vi "Controller Request Stop.vi"(7 "Sync Objects":T2, 8 "error in (no error)":errorcluster) -> (0 "error out":errorcluster)   [LabVIEW 2011, in "Controller VIs.lvlib"]
doc: "Requests the completion of all parallel loops running in the FOFB Controller. Sends a stop notification through the \"Stop Notifier\" and forces all blocking notifiers to be released."
uses:
  Controller VIs.lvlib
  Types Definitions/Type Synchronization Objects.ctl
  Types Definitions/Type Blocking Synchronization Objects.ctl
  Types Definitions/Type Monitoring Data.ctl
  Types Definitions/Type Operation Mode State.ctl
  Types Definitions/Type Diagnostics Data.ctl
  Types Definitions/Type CPU Loads Array.ctl
  Types Definitions/Type CPU Loads.ctl
  Types Definitions/Type Non-blocking Synchronization Objects.ctl
  Types Definitions/Type FOFB Variables.ctl
  Types Definitions/Type Actuation State.ctl
  Misc VIs.lvlib
  Type Definitions.lvlib
panel:
  out "Blocking":T1
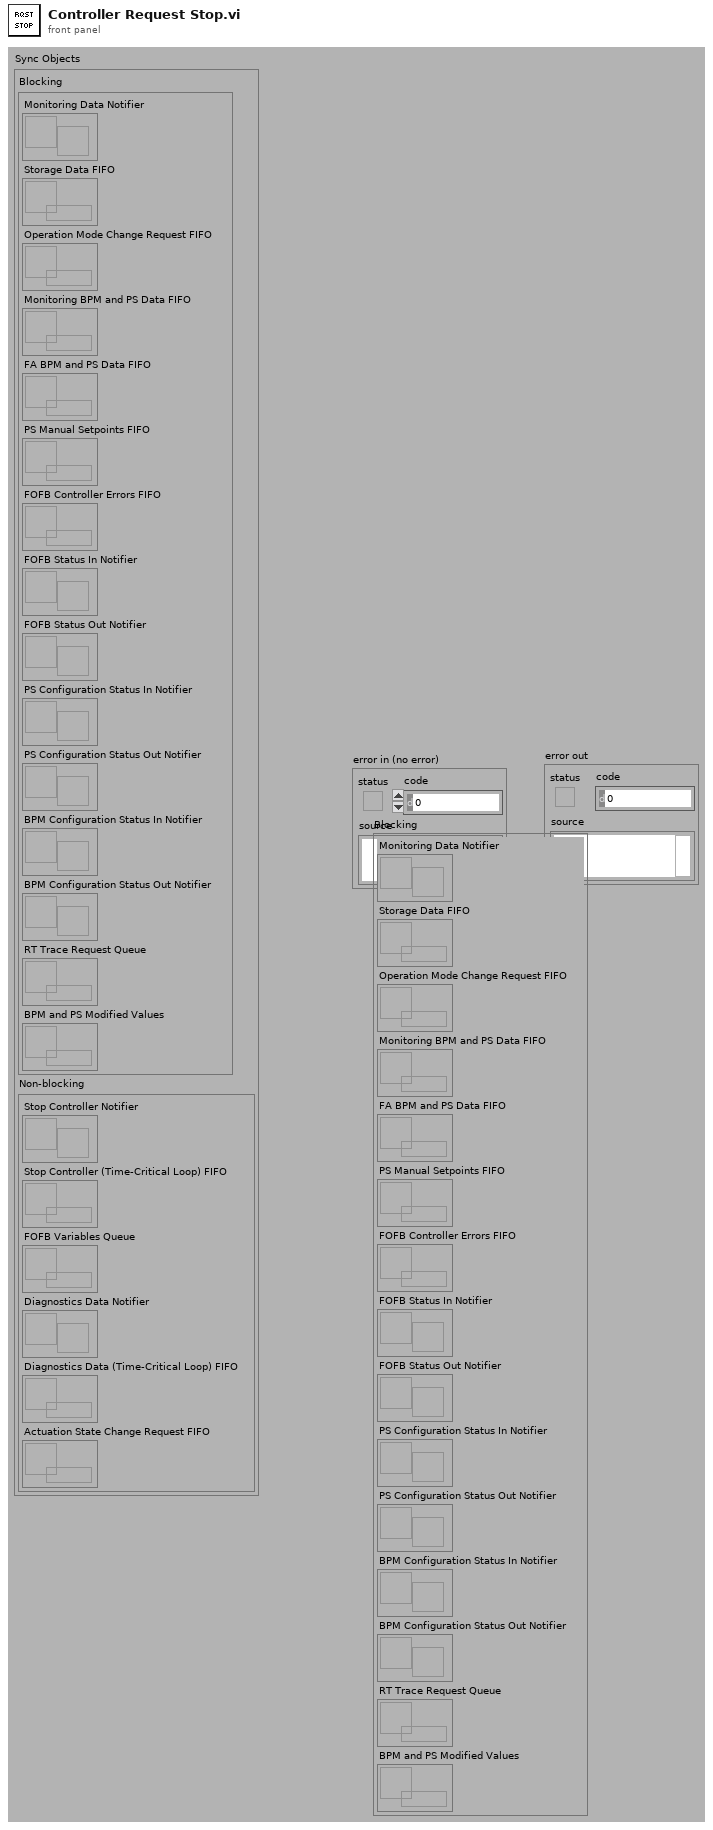
[diagram p1: front panel]
types:
  T1 = typedef "Type Definitions.lvlib/Type Blocking Synchronization Objects.ctl" = cluster{"Monitoring Data Notifier":refnum<notifier>, "Storage Data FIFO":refnum<queue>, "Operation Mode Change Request FIFO":refnum<k33>, "Monitoring BPM and PS Data FIFO":refnum<k33>, "FA BPM and PS Data FIFO":refnum<k33>, "PS Manual Setpoints FIFO":refnum<k33>, "FOFB Controller Errors FIFO ":refnum<k33>, "FOFB Status In Notifier":refnum<notifier>, "FOFB Status Out Notifier":refnum<notifier>, "PS Configuration Status In Notifier":refnum<notifier>, "PS Configuration Status Out Notifier":refnum<notifier>, "BPM Configuration Status In Notifier":refnum<notifier>, "BPM Configuration Status Out Notifier":refnum<notifier>, "RT Trace Request Queue":refnum<queue>, "BPM and PS Modified Values":refnum<k33>}
  T2 = typedef "Type Definitions.lvlib/Type Synchronization Objects.ctl" = cluster{"Blocking":T1, "Non-blocking":T3}
  T3 = typedef "Type Definitions.lvlib/Type Non-blocking Synchronization Objects.ctl" = cluster{"Stop Controller Notifier":refnum<notifier>, "Stop Controller (Time-Critical Loop) FIFO":refnum<k33>, "FOFB Variables Queue":refnum<queue>, "Diagnostics Data Notifier":refnum<notifier>, "Diagnostics Data (Time-Critical Loop) FIFO":refnum<k33>, "Actuation State Change Request FIFO":refnum<k33>}
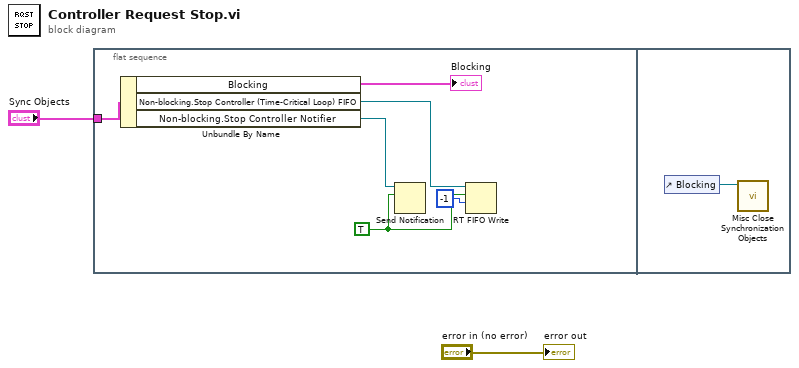
[diagram p0: block diagram]
diagram:
  n1 = flat-sequence {
    tunnel: "Sync Objects" -> [w8]
    frame #0 {
      w4 = TRUE ("notification")
      n2 = Unbundle By Name(w8) -> ("Blocking"=→"Blocking":T1, "Non-blocking.Stop Controller (Time-Critical Loop) FIFO"=w6:refnum<k33>, "Non-blocking.Stop Controller Notifier"=w7:refnum<notifier>)
      n3 = Send Notification(notification=w4, notifier=w7) -> ()  [unwired: 1 in, 2 out]
      n4 = RT FIFO Write(0:w6, 1:w4, 2:-1 ("timeout in ms (0)")) -> ()  [unwired: 2 in, 4 out]
    }
    frame #1 {
      n5 = control-ref of="Blocking"() -> (w9:refnum<vi>)
      n6 = call "Misc Close Synchronization Objects.vi"("Cluster Reference"=w9) -> ()  [unwired: 10 in, 1 out]
    }
  }
  "error out" <- "error in (no error)"
